vi "InitializeWatchdogMap.vi"(8 "error in (no error)":errorcluster) -> (0 "error out":errorcluster)   [LabVIEW 2017]
uses:
  <vilib>/addons/PointValueMap/subVIs/Point_Write_i32.vi
  <vilib>/addons/InsightCM/Utilities/GlobalConfiguration/GlobalConfiguration.lvlib
  <vilib>/addons/PointValueMap/PointValueMap.lvlib
  <vilib>/addons/InsightCM/Utilities/PropertyHelpers/PropertyHelpers.lvlib
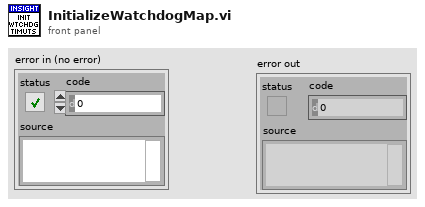
[diagram p1: front panel]
types:
  T1 = typedef "SectionKeyValues.ctl" = cluster{"Section":string, "KeyValues":T2[]}
  T2 = typedef "KeyValuePair.ctl" = cluster{"Key":string, "Value":string}
  T3 = typedef "PointValueMap.lvlib/PointMap.ctl" = refnum<data-value>
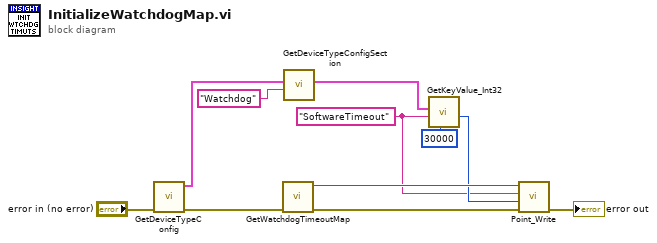
[diagram p0: block diagram]
diagram:
  w4 = "SoftwareTimeout" ("Tag")
  n1 = call <vilib>:"GetDeviceTypeConfig.vi"("error in (no error)"="error in (no error)") -> ("error out"=w9:errorcluster, "key values"=w10:T1[])  [unwired: 8 in, 1 out]
  n2 = call <vilib>:"GetWatchdogTimeoutMap.vi"("error in (no error)"=w9) -> ("error out"=w8:errorcluster, "WatchDogMap"=w7:T3)  [unwired: 9 in]
  n3 = call <vilib>:"GetDeviceTypeConfigSection.vi"("key"="Watchdog", "key values"=w10) -> ("key value pairs out"=w3:T2[])  [unwired: 8 in, 1 out]
  n4 = call <vilib>:"GetKeyValue_Int32.vi"("default"=30000, "key"=w4, "key value pairs"=w3) -> ("value"=w6:i32)  [unwired: 6 in, 2 out]
  n5 = call-poly <vilib>:"Point_Write.vi"("Error In"=w8, "Value"=w6, "Tag"=w4, "Map"=w7) -> ("Error Out"=→"error out":errorcluster)  [unwired: 6 in, 1 out]
